vi "MonitorVI.vi"(11 "Input":cluster{"stop":refnum<vi>, "numeric":refnum<vi>}) -> ()   [LabVIEW 2011]
panel:
  out "Waveform Chart":dbl(graph)
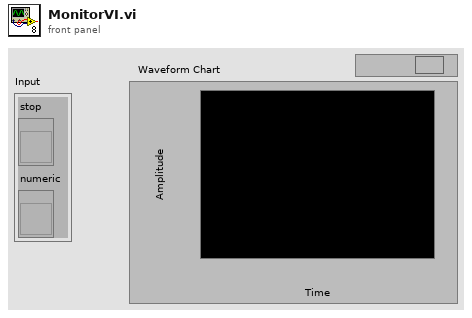
[diagram p1: front panel]
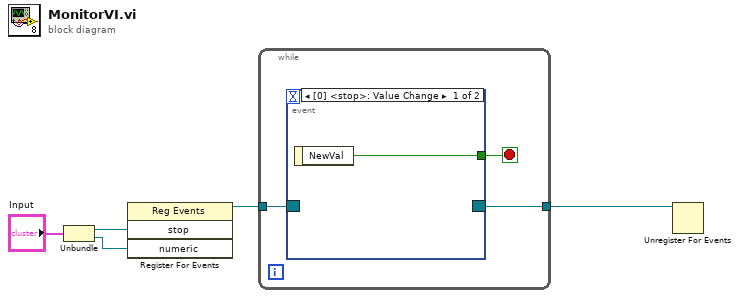
[diagram p0: block diagram]
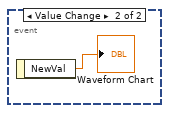
[diagram p2: hidden frame]
diagram:
  n1 = Unbundle("Input") -> ("stop"=w3:refnum<vi>, "numeric"=w2:refnum<vi>)
  n2 = register-events(w3, w2) -> (reference out=w1:refnum<event-registration>)  [unwired: 2 in, 1 out]
  n3 = while {
    tunnel: [w8] -> w5
    tunnel: w1 -> [w7]
    stop <- w6 stop-if-true
    n4 = event shown="[0] <stop>: Value Change" {
      selector: w7 -> [_ _]
      dyn-events: [_ _] -> w8
      timeout: _ -> [_ _]
      tunnel: [w9 _] -> w6
      event Value Change {
        n5 = event-data() -> ("NewVal"=w9:bool)  [unwired: 1 in]
      }
      event Value Change {
        n6 = event-data() -> ("NewVal"=→"Waveform Chart":dbl)  [unwired: 1 in]
      }
    }
  }
  n7 = Unregister For Events(event registration refnum=w5) -> ()  [unwired: 1 in, 1 out]
